vi "constructor.vi"(8 "error in (no error)":errorcluster, 11 "deviceName":string) -> (0 "error out":errorcluster, 3 "AnalogOutput out":refnum<class "AnalogOutput.lvclass">)   [LabVIEW 2011, in "Hardware.lvlib" / "Channels.lvlib" / "AnalogOutput.lvclass"]
uses:
  AnalogOutput.lvclass
  niDAQmxAO.lvclass
  SoundAO/SoundAO.lvclass
  K2602/K2602.lvclass
  HamegHMPSupply/HamegHMPSupply.lvclass
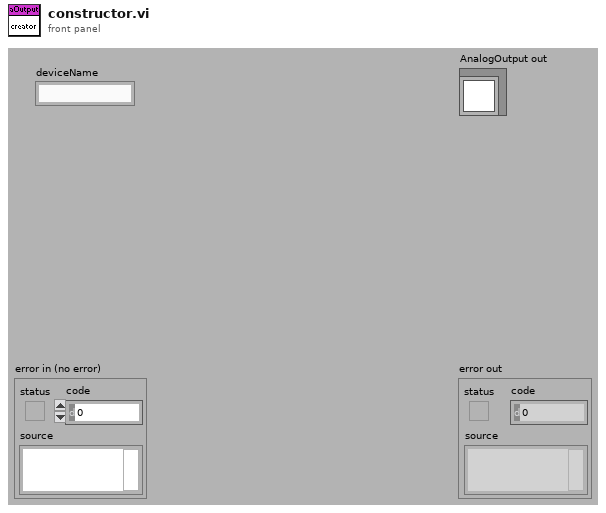
[diagram p1: front panel]
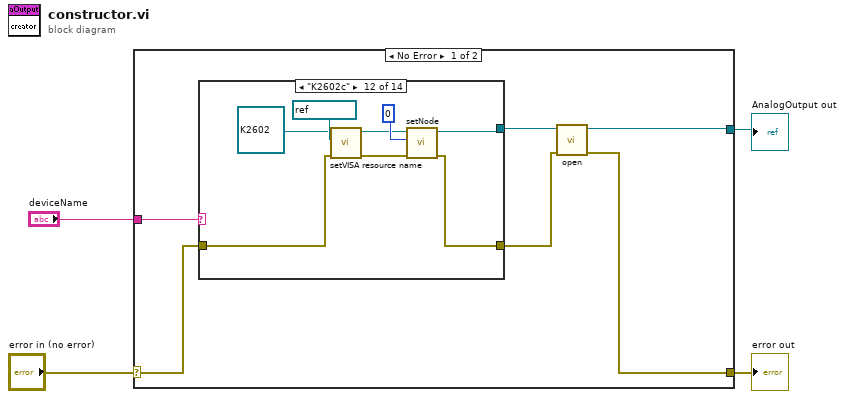
[diagram p0: block diagram]
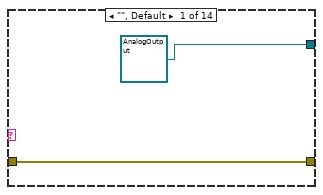
[diagram p2: hidden frame]
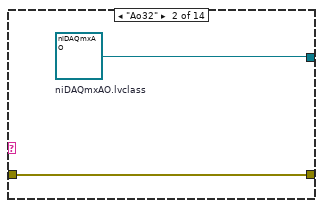
[diagram p3: hidden frame]
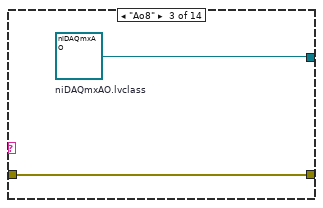
[diagram p4: hidden frame]
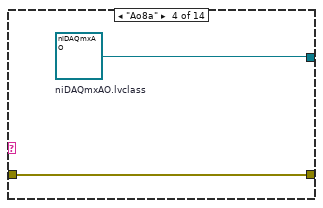
[diagram p5: hidden frame]
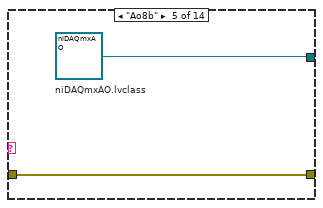
[diagram p6: hidden frame]
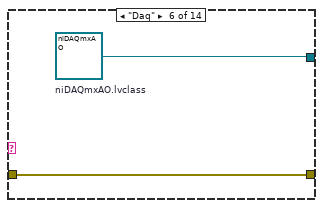
[diagram p7: hidden frame]
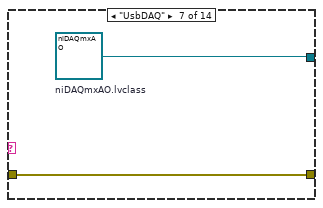
[diagram p8: hidden frame]
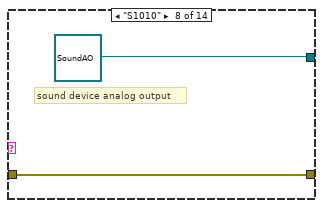
[diagram p9: hidden frame]
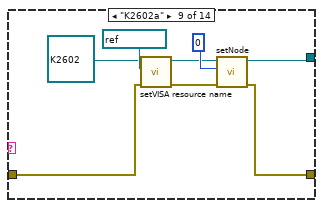
[diagram p10: hidden frame]
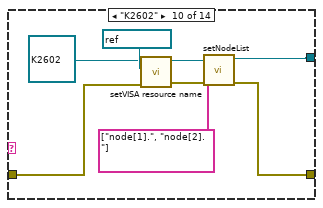
[diagram p11: hidden frame]
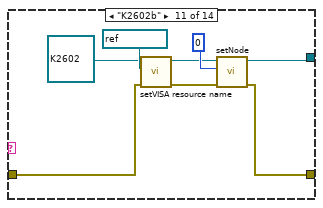
[diagram p12: hidden frame]
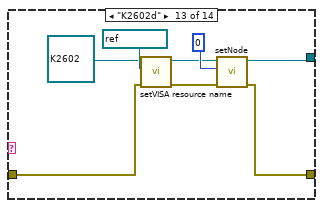
[diagram p13: hidden frame]
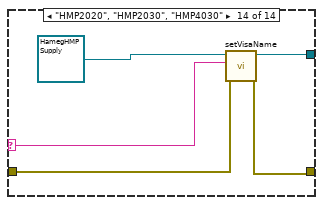
[diagram p14: hidden frame]
diagram:
  n1 = case shown="No Error" "error in (no error)" {
    selector: "error in (no error)" -> [w10 w72]
    tunnel: [w5 w72] -> w3
    tunnel: [w7 _] -> w2
    tunnel: "deviceName" -> [w9 _]
    frame No Error {
      n2 = case shown="\"K2602c\"" w9 {
        selector: w9 -> [_ _ _ _ _ _ _ _ _ _ _ _ _ w71]
        tunnel: [refnum<class "AnalogOutput.lvclass"> refnum ("Hardware:Channels.lvlib:AnalogOutput.lvclass") w13 w15 w17 w19 w21 w23 refnum<class "SoundAO.lvclass"> refnum ("Hardware:Channels.lvlib:SoundAO.lvclass") w28 w37 w44 w52 w60 w70] -> w8
        tunnel: w10 -> [w12 w14 w16 w18 w20 w22 w24 w26 w29 w40 w45 w53 w61 w67]
        tunnel: [w12 w14 w16 w18 w20 w22 w24 w26 w27 w36 w43 w51 w59 w69] -> w6
        frame "", Default {
        }
        frame "Ao32" {
          w13 = refnum<class "niDAQmxAO.lvclass"> refnum  # niDAQmxAO.lvclass
        }
        frame "Ao8" {
          w15 = refnum<class "niDAQmxAO.lvclass"> refnum  # niDAQmxAO.lvclass
        }
        frame "Ao8a" {
          w17 = refnum<class "niDAQmxAO.lvclass"> refnum  # niDAQmxAO.lvclass
        }
        frame "Ao8b" {
          w19 = refnum<class "niDAQmxAO.lvclass"> refnum  # niDAQmxAO.lvclass
        }
        frame "Daq" {
          w21 = refnum<class "niDAQmxAO.lvclass"> refnum  # niDAQmxAO.lvclass
        }
        frame "UsbDAQ" {
          w23 = refnum<class "niDAQmxAO.lvclass"> refnum  # niDAQmxAO.lvclass
        }
        frame "S1010" {
          # "sound device analog output"
        }
        frame "K2602a" {
          n3 = call "setVISA resource name.vi"("error in (no error)"=w29, "VISA resource name"=refnum<visa-resource-name> "k2602a", "K2602 in"=refnum<class "K2602.lvclass"> refnum ("Hardware:Channels.lvlib:K2602.lvclass")) -> ("error out"=w33:errorcluster, "K2602 out"=w31:refnum<class "K2602.lvclass">)  [unwired: 7 in]
          n4 = call "setNode.vi"("error in (no error)"=w33, "node"=0, "K2602 in"=w31) -> ("error out"=w27:errorcluster, "K2602 out"=w28:refnum<class "K2602.lvclass">)  [unwired: 7 in]
        }
        frame "K2602" {
          n5 = call "setVISA resource name.vi"("error in (no error)"=w40, "VISA resource name"=refnum<visa-resource-name> "keithley", "K2602 in"=refnum<class "K2602.lvclass"> refnum ("Hardware:Channels.lvlib:K2602.lvclass")) -> ("error out"=w38:errorcluster, "K2602 out"=w39:refnum<class "K2602.lvclass">)  [unwired: 7 in]
          n6 = call "setNodeList.vi"("error in (no error)"=w38, "nodeList"=string[] ["node[1].", "node[2]."], "K2602 in"=w39) -> ("error out"=w36:errorcluster, "K2602 out"=w37:refnum<class "K2602.lvclass">)  [unwired: 7 in]
        }
        frame "K2602b" {
          n7 = call "setVISA resource name.vi"("error in (no error)"=w45, "VISA resource name"=refnum<visa-resource-name> "k2602b", "K2602 in"=refnum<class "K2602.lvclass"> refnum ("Hardware:Channels.lvlib:K2602.lvclass")) -> ("error out"=w49:errorcluster, "K2602 out"=w47:refnum<class "K2602.lvclass">)  [unwired: 7 in]
          n8 = call "setNode.vi"("error in (no error)"=w49, "node"=0, "K2602 in"=w47) -> ("error out"=w43:errorcluster, "K2602 out"=w44:refnum<class "K2602.lvclass">)  [unwired: 7 in]
        }
        frame "K2602c" {
          n9 = call "setVISA resource name.vi"("error in (no error)"=w53, "VISA resource name"=refnum<visa-resource-name> "k2602c", "K2602 in"=refnum<class "K2602.lvclass"> refnum ("Hardware:Channels.lvlib:K2602.lvclass")) -> ("error out"=w57:errorcluster, "K2602 out"=w55:refnum<class "K2602.lvclass">)  [unwired: 7 in]
          n10 = call "setNode.vi"("error in (no error)"=w57, "node"=0, "K2602 in"=w55) -> ("error out"=w51:errorcluster, "K2602 out"=w52:refnum<class "K2602.lvclass">)  [unwired: 7 in]
        }
        frame "K2602d" {
          n11 = call "setVISA resource name.vi"("error in (no error)"=w61, "VISA resource name"=refnum<visa-resource-name> "k2602d", "K2602 in"=refnum<class "K2602.lvclass"> refnum ("Hardware:Channels.lvlib:K2602.lvclass")) -> ("error out"=w65:errorcluster, "K2602 out"=w63:refnum<class "K2602.lvclass">)  [unwired: 7 in]
          n12 = call "setNode.vi"("error in (no error)"=w65, "node"=0, "K2602 in"=w63) -> ("error out"=w59:errorcluster, "K2602 out"=w60:refnum<class "K2602.lvclass">)  [unwired: 7 in]
        }
        frame "HMP2020", "HMP2030", "HMP4030" {
          n13 = call "setVisaName.vi"("error in (no error)"=w67, "name"=w71, "HamegHMPSupply in"=refnum<class "HamegHMPSupply.lvclass"> refnum) -> ("error out"=w69:errorcluster, "HamegHMPSupply out"=w70:refnum<class "HamegHMPSupply.lvclass">)  [unwired: 7 in]
        }
      }
      n14 = call-dynamic "open.vi"("error in (no error)"=w6, "AnalogOutput in"=w8) -> ("error out"=w5:errorcluster, "AnalogOutput out"=w7:refnum<class "AnalogOutput.lvclass">)  [unwired: 8 in]
    }
    frame Error {
    }
  }
  "error out" <- w3
  "AnalogOutput out" <- w2
